vi "PLL_PID.vi"(8 "error in (no error)":errorcluster, 9 "REF []":waveform(dbl), 10 "AO []":waveform(dbl), 11 "LockinDAQ in":refnum<class "Lockin.DAQ.lvclass">) -> (0 "error out":errorcluster, 1 "phase output (°)":dbl, 2 "frequency output (Hz)":dbl, 3 "LockinDAQ out":refnum<class "Lockin.DAQ.lvclass">)   [LabVIEW 2016, in "Lockin.DAQ.lvclass"]
doc: "Please ensure that at least one period is generated or else the measurement VIs do not work properly."
uses:
  Lockin.DAQ.lvclass
  <vilib>/Waveform/WDTOps.llb/WDT Waveform Duration DBL.vi
  <vilib>/addons/control/pid/pid.llb/PID (DBL).vi
  <vilib>/measure/matone.llb/Extract Single Tone Information 1 Chan.vi
  <vilib>/Analysis/NI_AALPro.lvlib
  <vilib>/addons/control/pid/NI_PID_pid.lvlib
  <vilib>/measure/NI_MAPro.lvlib
  <vilib>/ptbypt/NI_PtbyPt.lvlib
panel:
  out "Phase Chart":cluster{dbl, "output":dbl}(graph)
  out "Frequency Chart":T1(graph)
  out "process frequency":dbl format="%.2p"
  out "detected frequency (set point)":dbl format="%.2p"
  in  "PID_Phase":T2={"proportional gain (Kc)"=0.1, "integral time (Ti, min)"=0.0008, "derivative time (Td, min)"=0.0} {"derivative time (Td, min)" format="%.3f"; "integral time (Ti, min)" items=["Take a Coffee"=0.1, "Yawning"=0.01, "Take a Deep Breath"=0.001, "Normal"=0.0008, "A Little Bit Fast"=0.0001, "Fast"=1e-05, "Too Fast"=1e-06]; "proportional gain (Kc)" format="%.3f"}
  in  "PID_Frequency":T2={"proportional gain (Kc)"=0.9, "integral time (Ti, min)"=0.0008, "derivative time (Td, min)"=0.0} {"derivative time (Td, min)" format="%.3f"; "integral time (Ti, min)" items=["Take a Coffee"=0.1, "Yawning"=0.01, "Take a Deep Breath"=0.001, "Normal"=0.0008, "A Little Bit Fast"=0.0001, "Fast"=1e-05, "Too Fast"=1e-06]; "proportional gain (Kc)" format="%.3f"}
  out "Waveform Graph":waveform(dbl)[](graph)=[{"t0"=timestamp(0 s since 1904-01-01), "dt"=0.001, "Y"=array[1000 elements]}, {"t0"=timestamp(0 s since 1904-01-01), "dt"=0.001, "Y"=array[1000 elements]}]
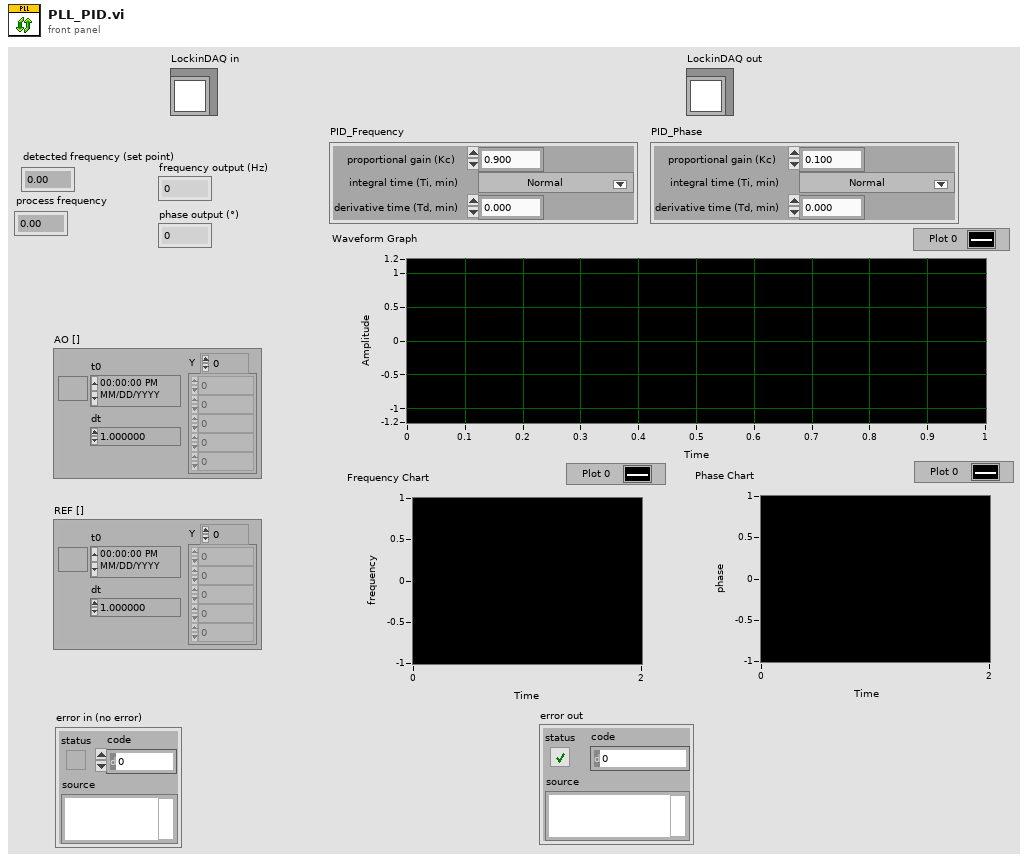
[diagram p1: front panel]
types:
  T1 = cluster{"detected frequency":dbl, "detected frequency":dbl, "output":dbl}
  T2 = cluster{"proportional gain (Kc)":dbl, "integral time (Ti, min)":dbl, "derivative time (Td, min)":dbl}
  T3 = cluster{"detected frequency":dbl, "detected frequency":dbl, "output":dbl}[]
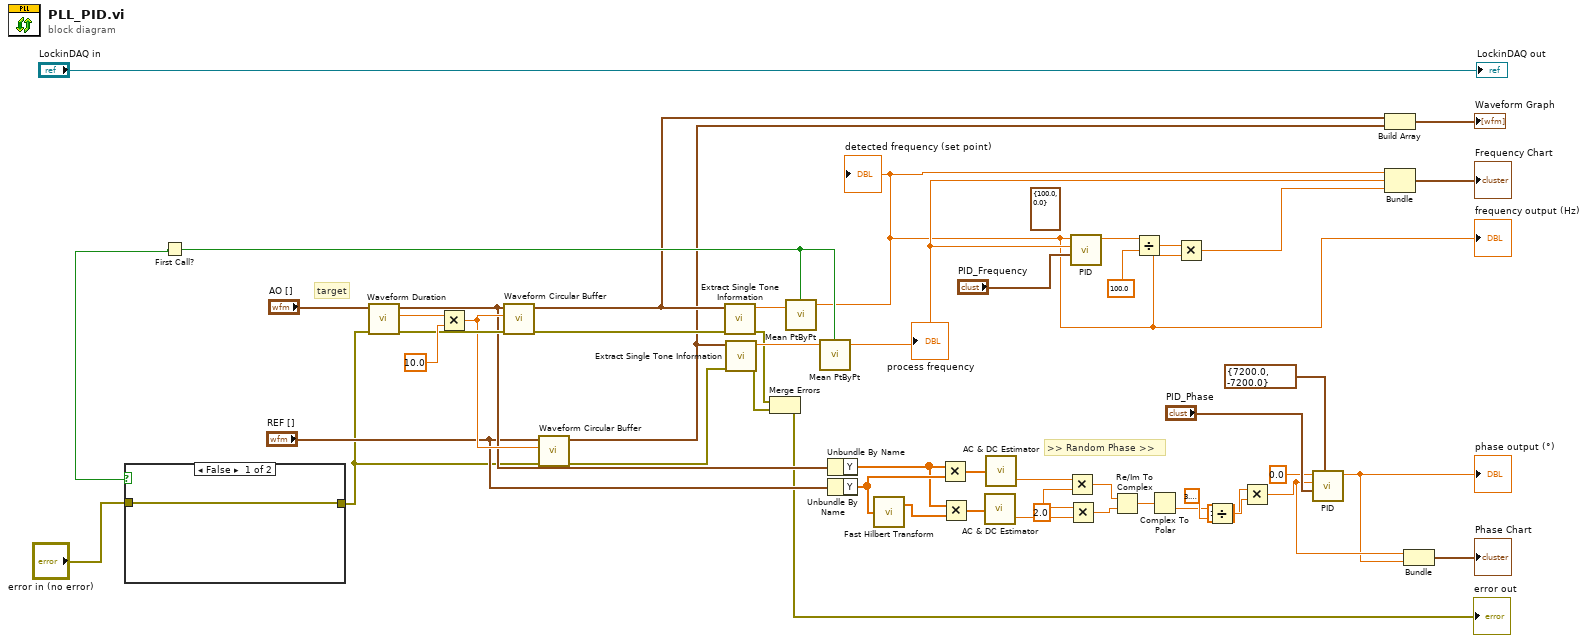
[diagram p0: block diagram]
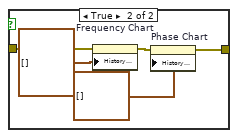
[diagram p2: hidden frame]
diagram:
  (unwired) cluster{"output high":dbl, "output low":dbl} {"output high"=100.0, "output low"=0.0} ("output range")
  w35 = 2.0 ("x")
  # "target"
  # ">> Random Phase >>"
  n1 = First Call?() -> (First Call?: T/F=w18:bool)
  n2 = case shown="False" w18 {
    tunnel: [w51 w53] -> w5
    tunnel: "error in (no error)" -> [w51 w52]
    frame False {
    }
    frame True {
      n3 = property on="Frequency Chart" class="WFChart (strict)"(error in=w52, "History Data"=T3 []) -> (error out=w56:errorcluster)  [unwired: 1 in, 1 out]
      n4 = property on="Phase Chart" class="WFChart (strict)"(error in=w56, "History Data"=cluster{dbl, "output":dbl}[] []) -> (error out=w53:errorcluster)  [unwired: 1 in, 1 out]
    }
  }
  n5 = call-poly <vilib>:"Waveform Duration.vi"("error in (no error)"=w5, "waveform in"="AO []") -> ("error out"=w27:errorcluster, "duration"=w30:dbl, "waveform out"=w10:waveform(dbl))  [unwired: 7 in]
  n6 = Multiply(x=w30, y=10.0) -> (x*y=w24:dbl)
  n7 = call "Waveform Circular Buffer.vi"("error in"=w27, "buffer duration (s)"=w24, "waveform in"=w10) -> ("error out"=w26:errorcluster, "waveform out"=w16:waveform(dbl))  [unwired: 7 in]
  n8 = call "Waveform Circular Buffer.vi"("error in"=w5, "buffer duration (s)"=w24, "waveform in"="REF []") -> ("error out"=w4:errorcluster, "waveform out"=w11:waveform(dbl))  [unwired: 7 in]
  n9 = call-poly <vilib>:"Extract Single Tone Information.vi"("error in (no error)"=w26, "time signal in"=w16) -> ("error out"=w3:errorcluster, "detected frequency"=w19:dbl)  [unwired: 4 in, 4 out]
  n10 = call-poly <vilib>:"Extract Single Tone Information.vi"("error in (no error)"=w4, "time signal in"=w11) -> ("error out"=w2:errorcluster, "detected frequency"=w23:dbl)  [unwired: 4 in, 4 out]
  n11 = Merge Errors(w3, w2) -> (→"error out":errorcluster)
  n12 = call <vilib>:"Mean PtByPt.vi"("x"=w19, "initialize"=w18) -> ("mean"=w7:dbl)  [unwired: 2 in, 1 out]
  "frequency output (Hz)" <- w7
  "detected frequency (set point)" <- w7
  n13 = call <vilib>:"Mean PtByPt.vi"("x"=w23, "initialize"=w18) -> ("mean"=w17:dbl)  [unwired: 2 in, 1 out]
  "process frequency" <- w17
  n14 = Unbundle By Name(w10) -> ("Y"=w47:dbl[])
  n15 = Unbundle By Name("REF []") -> ("Y"=w49:dbl[])
  n16 = call <vilib>:"Fast Hilbert Transform.vi"("X"=w49) -> ("Hilbert{X}"=w48:dbl[])  [unwired: 1 out]
  n17 = Multiply(x=w47, y=w49) -> (x*y=w46:dbl[])
  n18 = Multiply(x=w47, y=w48) -> (x*y=w45:dbl[])
  n19 = call <vilib>:"AC & DC Estimator.vi"("Signal (V)"=w45) -> ("DC estimate (V)"=w44:dbl)  [unwired: 1 out]
  n20 = call <vilib>:"AC & DC Estimator.vi"("Signal (V)"=w46) -> ("DC estimate (V)"=w36:dbl)  [unwired: 1 out]
  n21 = Multiply(x=w36, y=w35) -> (x*y=w38:dbl)
  n22 = Multiply(x=w35, y=w44) -> (x*y=w37:dbl)
  n23 = call-poly <vilib>:"PID.vi"("PID gains"="PID_Frequency", "process variable"=w17, "setpoint"=w7) -> ("output"=w20:dbl)  [unwired: 7 in, 1 out]
  n24 = Re/Im To Complex(1:w37, 2:w38) -> (0:w39:cdb)
  n25 = Divide(x=w20, y=100.0) -> (x/y=w21:dbl)
  n26 = Complex To Polar(r * e^(i*theta)=w39) -> (theta=w40:dbl)  [unwired: 1 out]
  n27 = Multiply(x=w21, y=w7) -> (x*y=w8:dbl)
  n28 = Divide(x=w40, y=3.141592653589793) -> (x/y=w42:dbl)
  n29 = Multiply(x=w42, y=180.0) -> (x*y=w14:dbl)
  n30 = call-poly <vilib>:"PID.vi"("output range"=cluster{"output high":dbl, "output low":dbl} {"output high"=7200.0, "output low"=-7200.0}, "PID gains"="PID_Phase", "process variable"=w14, "setpoint"=0.0) -> ("output"=w13:dbl)  [unwired: 6 in, 1 out]
  "phase output (°)" <- w13
  n31 = Build Array(w16, w11) -> (→"Waveform Graph":waveform(dbl)[])
  n32 = Bundle("mean"=w7, "mean"=w17, w8) -> (→"Frequency Chart":cluster{"mean":dbl, "mean":dbl, dbl})  [unwired: 1 in]
  n33 = Bundle(w14, "output"=w13) -> (→"Phase Chart":cluster{dbl, "output":dbl})  [unwired: 1 in]
  "LockinDAQ out" <- "LockinDAQ in"
